vi "EDS test 02.vi"() -> ()   [LabVIEW 2020]
panel:
  out "max value":dbl
  in  "Ultrasonic 01":dbl
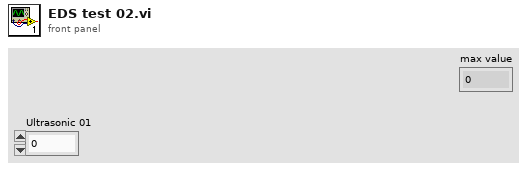
[diagram p1: front panel]
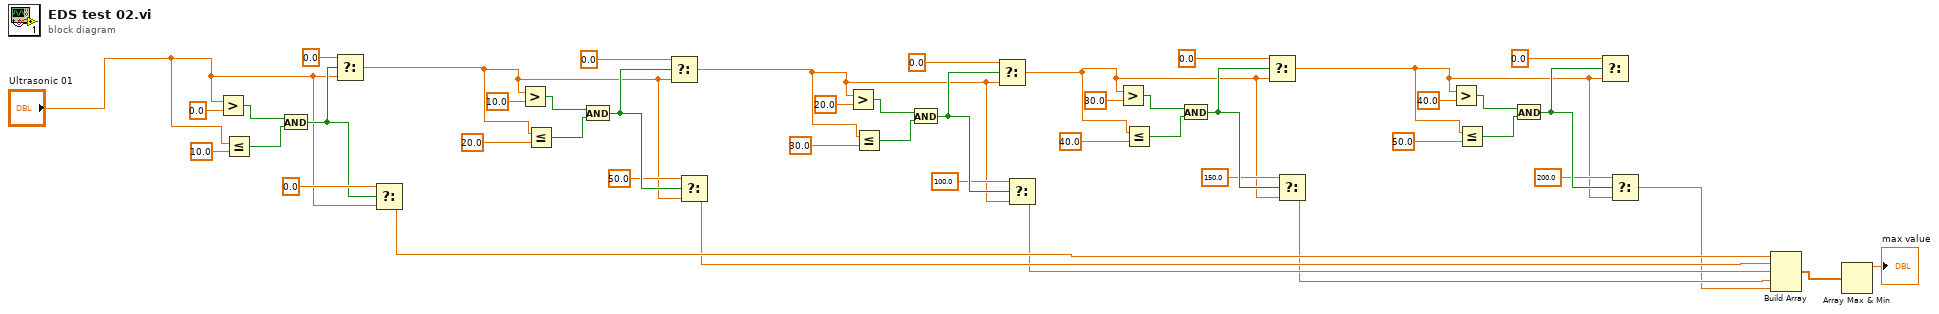
[diagram p0: block diagram]
diagram:
  n1 = Greater?(x="Ultrasonic 01", y=0.0) -> (0:w45:bool)
  n2 = Less Or Equal?(x="Ultrasonic 01", y=10.0) -> (x <= y?=w44:bool)
  n3 = And(x=w45, y=w44) -> (x .and. y?=w37:bool)
  n4 = Select(t=0.0, s=w37, f="Ultrasonic 01") -> (s? t:f=w33:dbl)
  n5 = Select(t=0.0, s=w37, f="Ultrasonic 01") -> (s? t:f=w7:dbl)
  n6 = Greater?(x=w33, y=10.0) -> (0:w41:bool)
  n7 = Less Or Equal?(x=w33, y=20.0) -> (x <= y?=w40:bool)
  n8 = And(x=w41, y=w40) -> (x .and. y?=w35:bool)
  n9 = Select(t=0.0, s=w35, f=w33) -> (s? t:f=w25:dbl)
  n10 = Select(t=50.0, s=w35, f=w33) -> (s? t:f=w6:dbl)
  n11 = Greater?(x=w25, y=20.0) -> (0:w30:bool)
  n12 = Less Or Equal?(x=w25, y=30.0) -> (x <= y?=w29:bool)
  n13 = And(x=w30, y=w29) -> (x .and. y?=w27:bool)
  n14 = Select(t=0.0, s=w27, f=w25) -> (s? t:f=w17:dbl)
  n15 = Select(t=100.0, s=w27, f=w25) -> (s? t:f=w5:dbl)
  n16 = Greater?(x=w17, y=30.0) -> (0:w22:bool)
  n17 = Less Or Equal?(x=w17, y=40.0) -> (x <= y?=w21:bool)
  n18 = And(x=w22, y=w21) -> (x .and. y?=w19:bool)
  n19 = Select(t=0.0, s=w19, f=w17) -> (s? t:f=w9:dbl)
  n20 = Select(t=150.0, s=w19, f=w17) -> (s? t:f=w4:dbl)
  n21 = Greater?(x=w9, y=40.0) -> (0:w14:bool)
  n22 = Less Or Equal?(x=w9, y=50.0) -> (x <= y?=w13:bool)
  n23 = And(x=w14, y=w13) -> (x .and. y?=w11:bool)
  n24 = Select(t=0.0, s=w11, f=w9) -> ()  [unwired: 1 out]
  n25 = Select(t=200.0, s=w11, f=w9) -> (s? t:f=w3:dbl)
  n26 = Build Array(w7, w6, w5, w4, w3) -> (w2:dbl[])
  n27 = Array Max & Min(array=w2) -> (max value=→"max value":dbl)  [unwired: 3 out]
